vi "viserver.vi"(11 "args":T1) -> (0 "error out":errorcluster)   [LabVIEW 2013]
uses:
  executables/arguments.ctl
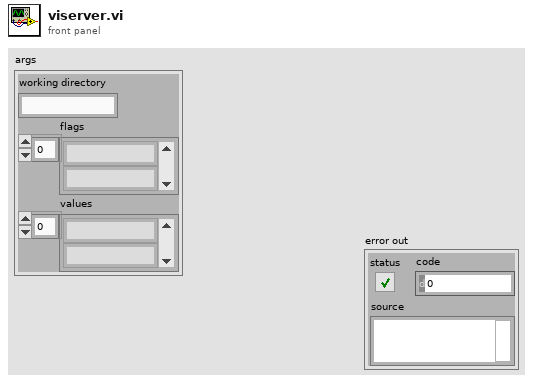
[diagram p1: front panel]
types:
  T1 = typedef "arguments.ctl" = cluster{"working directory":string, "flags":string[], "values":string[]}
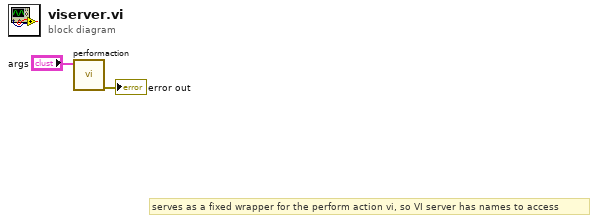
[diagram p0: block diagram]
diagram:
  # "serves as a fixed wrapper for the perform action vi, so VI server has names to access"
  n1 = call "performaction.vi"("command line arguments"="args") -> ("error out"=→"error out":errorcluster)  [unwired: 10 in]
